vi "WPI_SPIOpen.vi"(6 "Chip Select Active High (F)":bool, 8 "error in":errorcluster, 9 "Mode (3)":T1=enum."Mode 3 (Clk Idle High,Sample on Trailing)", 10 "Clock Rate (Hz)":dbl=500000.0, 11 "SPI Bus":T2=enum."Invalid") -> (0 "error out":errorcluster, 3 "SPIDevRef":T3={"DevStatus"={"status"=FALSE, "code"=0, "source"=""}, "Handle"=0, "SPI Bus"=enum."Invalid"})   [LabVIEW 2017]
doc: "Opens a reference to the SPI Engine. You must open a reference before using any other VIs on this palette. After you open a reference to the SPI Engine, you can use the other SPI VIs to access and monitor the sensors or custom circuits from the SPI Engine.\n\nThis software is licensed. Open the labview\\readme\\WPI Robotics Library Open Source License.txt file for more information."
uses:
  <vilib>/Rock Robotics/WPI/SPI/WPI_SPIDevRef.ctl
  <vilib>/Rock Robotics/SystemInterfaces/spilib/spi_bus.ctl
  <vilib>/Rock Robotics/WPI/SPI/WPI_SPIMode.ctl
  <vilib>/Rock Robotics/WPI/SPI/WPI_SPIBusCacheOp.ctl
  <vilib>/Rock Robotics/SystemInterfaces/NetworkCommunication/NetComm_UsageReport_ResourceType.ctl
  <vilib>/Rock Robotics/SystemInterfaces/DIO/FPGA_DIOChannel.ctl
  <vilib>/Rock Robotics/SystemInterfaces/System/FPGA_SystemGet.vi
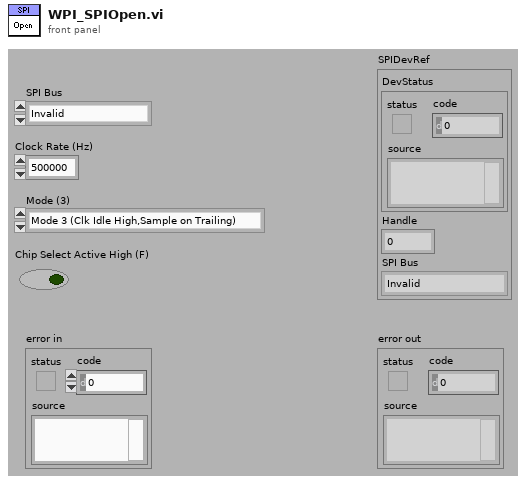
[diagram p1: front panel]
types:
  T1 = typedef "WPI_SPIMode.ctl" = enum16{"Mode 0 (Clk Idle Low,Sample on Leading)", "Mode 1 (Clk Idle Low,Sample on Trailing)", "Mode 2 (Clk Idle High,Sample on Leading)", "Mode 3 (Clk Idle High,Sample on Trailing)"}
  T2 = typedef "spi_bus.ctl" = enum16{"SPI On-Board, CS0", "SPI On-Board, CS1", "SPI On-Board, CS2", "SPI On-Board, CS3", "SPI MXP", "Invalid"}
  T3 = typedef "WPI_SPIDevRef.ctl" = cluster{"DevStatus":errorcluster, "Handle":i32, "SPI Bus":T2}
  T4 = typedef "WPI_SPIBusCacheOp.ctl" = enum16{"Acquire", "Release", "Status"}
  T5 = typedef "NetComm_UsageReport_ResourceType.ctl" = enum8{"Controller", "Module", "Language", "CANPlugin", "Accelerometer", "ADXL345", "AnalogChannel", "AnalogTrigger", "AnalogTriggerOutput", "CANJaguar", "Compressor", "Counter", "Dashboard", "DigitalInput", "DigitalOutput", "DriverStationCIO", "DriverStationEIO", "DriverStationLCD", "Encoder", "GearTooth", "Gyro", "I2C", "Framework", "Jaguar", "Joystick", "Kinect", "KinectStick", "PIDController", "Preferences", "PWM", "Relay", "RobotDrive", "SerialPort", "Servo", "Solenoid", "SPI", "Task", "Ultrasonic", "Victor", "Button", "Command", "AxisCamera", "PCVideoServer", "SmartDashboard", "Talon", "HiTechnicColorSensor", "HiTechnicAccel", "HiTechnicCompass", "SRF08", "AnalogOutput", "Victor SP", "Talon SRX", "CAN Talon SRX", "ADXL362 Accel", "ADXRS450 Gyro", "Rev SPARK", "Mindsensors SD540", "Digital Filter", "ADIS16448", "PDP", "PCM", "PigeonIMU", "Nidec Brushless", "CTRE CANifier", "CTRE Future 0", "CTRE Future 1", "CTRE Future 2", "CTRE Future 3", "CTRE Future 4", "CTRE Future 5", "CTRE Future 6"}
  T6 = typedef "FPGA_DIOChannel.ctl" = enum8{"DIO 0", "DIO 1", "DIO 2", "DIO 3", "DIO 4", "DIO 5", "DIO 6", "DIO 7", "DIO 8", "DIO 9", "DIO MXP 0", "DIO MXP 1", "DIO MXP 2", "DIO MXP 3", "DIO MXP 4", "DIO MXP 5", "DIO MXP 6", "DIO MXP 7", "DIO MXP 8", "DIO MXP 9", "DIO MXP 10", "DIO MXP 11", "DIO MXP 12", "DIO MXP 13", "DIO MXP 14", "DIO MXP 15", "SPI Port CS1", "SPI Port CS2", "SPI Port CS3", "SPI Port MISO", "SPI Port MOSI", "Invalid"}
  T7 = typedef "FPGA_DIODevRef.ctl" = cluster{"DevStatus":errorcluster}
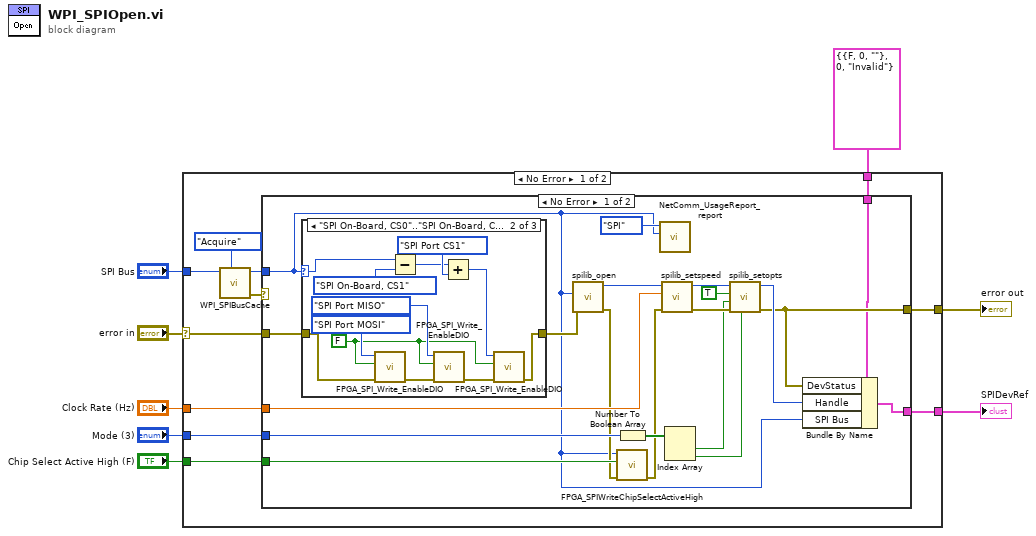
[diagram p0: block diagram]
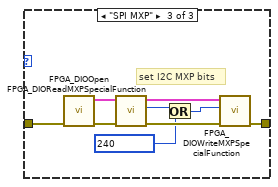
[diagram p3: hidden frame]
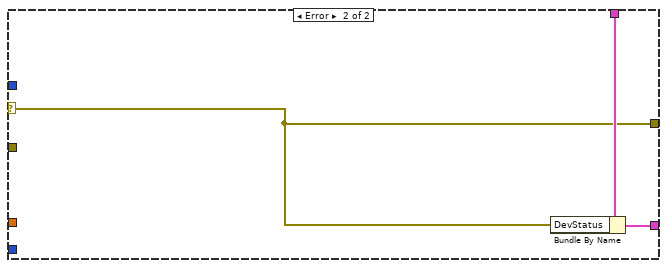
[diagram p4: hidden frame]
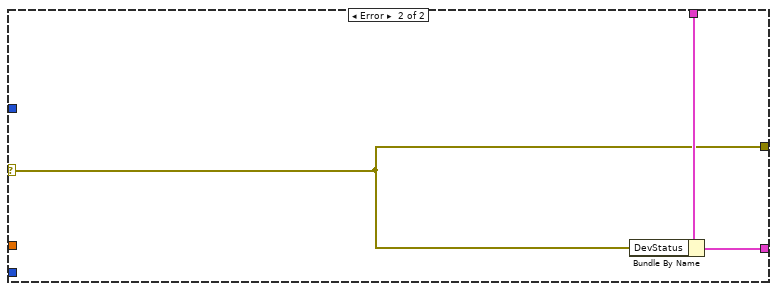
[diagram p5: hidden frame]
diagram:
  n1 = case shown="No Error" "error in" {
    selector: "error in" -> [w15 w66]
    tunnel: [w17 w66] -> w8
    tunnel: "SPI Bus" -> [w14 _]
    tunnel: "Clock Rate (Hz)" -> [w19 _]
    tunnel: "Mode (3)" -> [w18 _]
    tunnel: "Chip Select Active High (F)" -> [w16 _]
    tunnel: T3 {"DevStatus"={"status"=FALSE, "code"=0, "source"=""}, "Handle"=0, "SPI Bus"=enum."Invalid"} ("SPIDevRef") -> [w10 w67]
    tunnel: [w9 w65] -> w1
    frame No Error {
      n2 = call <vilib>:"WPI_SPIBusCache.vi"("Operation"=WPI_SPIBusCacheOp."Acquire", "SPI Bus"=w14) -> ("error out"=w12:errorcluster, "SPI Bus Allocated"=w13:T2)  [unwired: 7 in, 1 out]
      n3 = case shown="No Error" w12 {
        selector: w12 -> [_ w62]
        tunnel: w19 -> [w37 _]
        tunnel: w18 -> [w34 _]
        tunnel: [w25 w62] -> w17
        tunnel: w16 -> [w31 _]
        tunnel: w15 -> [w28 _]
        tunnel: w13 -> [w24 _]
        tunnel: w10 -> [w23 w64]
        tunnel: [w22 w63] -> w9
        frame No Error {
          n4 = case shown="\"SPI On-Board, CS0\"..\"SPI On-Board, CS3\"" w24 {
            selector: w24 -> [_ w52 _]
            tunnel: w28 -> [w40 w44 w56]
            tunnel: [w40 w47 w55] -> w27
            frame Default {
            }
            frame "SPI On-Board, CS0".."SPI On-Board, CS3" {
              w41 = FALSE ("Enable DIO (F)")
              n5 = call <vilib>:"FPGA_SPI_Write_EnableDIO.vi"("error in (no error)"=w44, "Enable DIO (F)"=w41, "DIOChannel"=FPGA_DIOChannel."SPI Port MOSI" ("DIO Channel")) -> ("error out"=w45:errorcluster)  [unwired: 8 in]
              n6 = Subtract(x=w52, y=spi_bus."SPI On-Board, CS1" ("SPI Bus")) -> (x-y=w49:u16)
              n7 = call <vilib>:"FPGA_SPI_Write_EnableDIO.vi"("error in (no error)"=w45, "Enable DIO (F)"=w41, "DIOChannel"=FPGA_DIOChannel."SPI Port MISO" ("DIO Channel")) -> ("error out"=w46:errorcluster)  [unwired: 8 in]
              n8 = Add(x=w49, y=FPGA_DIOChannel."SPI Port CS1" ("DIO Channel")) -> (x+y=w48:u16)
              n9 = call <vilib>:"FPGA_SPI_Write_EnableDIO.vi"("error in (no error)"=w46, "Enable DIO (F)"=w41, "DIOChannel"=w48) -> ("error out"=w47:errorcluster)  [unwired: 8 in]
            }
            frame "SPI MXP" {
              # "set I2C MXP bits"
              n10 = call <vilib>:"FPGA_DIOOpen.vi"("error in (no error)"=w56) -> ("error out"=w60:errorcluster, "DIODeviceRef"=w61:T7)  [unwired: 1 in, 8 out]
              n11 = call <vilib>:"FPGA_DIOReadMXPSpecialFunction.vi"("error in (no error)"=w60, "DIODeviceRef In"=w61) -> ("error out"=w54:errorcluster, "EnableSpecialFunction"=w58:u16, "DIODeviceRef Out"=w59:T7)  [unwired: 7 in]
              n12 = Or(x=w58, y=u16 240 ("EnableSpecialFunction")) -> (x .or. y?=w57:u16)
              n13 = call <vilib>:"FPGA_DIOWriteMXPSpecialFunction.vi"("error in (no error)"=w54, "EnableSpecialFunction"=w57, "DIODeviceRef In"=w59) -> ("error out"=w55:errorcluster)  [unwired: 7 in, 1 out]
            }
          }
          n14 = call <vilib>:"spilib_open.vi"("error in (no error)"=w27, "SPI Bus"=w24) -> ("error out"=w29:errorcluster, "handle out"=w38:i32)  [unwired: 8 in]
          n15 = call <vilib>:"FPGA_SPIWriteChipSelectActiveHigh.vi"("error in (no error)"=w29, "Chip Select Active High (F)"=w31, "SPI Bus"=w24) -> ("error out"=w30:errorcluster)  [unwired: 8 in]
          n16 = Number To Boolean Array(number=w34) -> (Boolean array=w33:bool[])
          n17 = call <vilib>:"NetComm_UsageReport_report.vi"("Instance Number"=w24, "Resource Type"=NetComm_UsageReport_ResourceType."SPI") -> ()  [unwired: 10 in]
          n18 = call <vilib>:"spilib_setspeed.vi"("error in (no error)"=w30, "speed"=w37, "handle"=w38) -> ("error out"=w35:errorcluster, "handle out"=w36:i32)  [unwired: 7 in]
          n19 = Index Array(array=w33) -> (element #1=w21:bool, element #2=w20:bool)  [unwired: 2 in]
          n20 = call <vilib>:"spilib_setopts.vi"("clk_idle_high"=w20, "error in (no error)"=w35, "sample_on_trailing"=w21, "msb_first"=TRUE, "handle"=w36) -> ("error out"=w25:errorcluster, "handle out"=w26:i32)  [unwired: 5 in]
          n21 = Bundle By Name(cluster=w23, "DevStatus"=w25, "Handle"=w26, "SPI Bus"=w24) -> (w22:T3)
        }
        frame Error {
          n22 = Bundle By Name(cluster=w64, "DevStatus"=w62) -> (w63:T3)
        }
      }
    }
    frame Error {
      n23 = Bundle By Name(cluster=w67, "DevStatus"=w66) -> (w65:T3)
    }
  }
  "error out" <- w8
  "SPIDevRef" <- w1
